vi "StoreUUTResult.vi"(8 "error in (no error)":errorcluster, 10 "Table name":string="TestResult", 11 "Result":T1 {"THD"."magnitude" format="%.2p"; "THD"."f0" format="%0.2p"; "THD"."df" format="%0.2p"}) -> (0 "error out":errorcluster={"status"=TRUE, "code"=1, "source"="DB Tools Validate Inputs.vi->DB Tools Insert Data.vi->StoreUUTResult.vi<ERR>Argument error. The table name given is blank."})   [LabVIEW 2014]
uses:
  <vilib>/addons/database/Connection.llb/DB Tools Open Connec (String).vi
  <vilib>/addons/database/NI_Database_API.lvlib
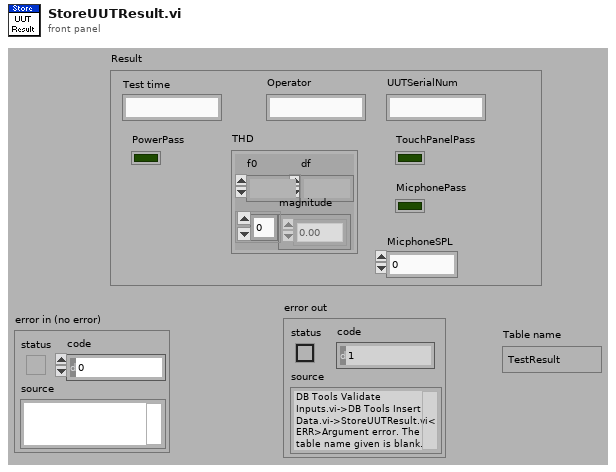
[diagram p1: front panel]
types:
  T1 = cluster{"Test time":string, "Operator":string, "UUTSerialNum":string, "PowerPass":bool, "THD":cluster{"f0":dbl, "df":dbl, "magnitude":dbl[]}, "TouchPanelPass":bool, "MicphonePass":bool, "MicphoneSPL":dbl}
  T2 = typedef "NI_Database_API.lvlib/Conn ObjectReference.ctl" = refnum<k1>
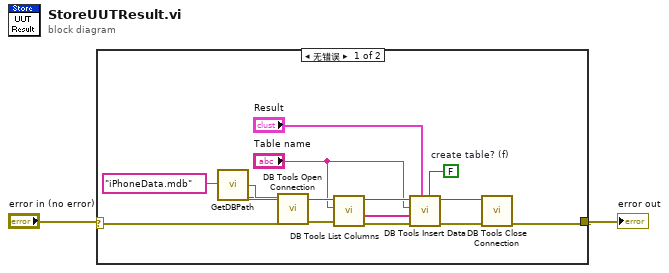
[diagram p0: block diagram]
diagram:
  n1 = case shown="无错误" "error in (no error)" {
    selector: "error in (no error)" -> [w12 w17]
    tunnel: [w11 w17] -> w1
    frame No Error {
      w10 = FALSE  # create table? (f)
      n2 = call "GetDBPath.vi"("Filename"="iPhoneData.mdb") -> ("Connection"=w14:string)
      n3 = call-poly <vilib>:"DB Tools Open Connection.vi"("error in (no error)"=w12, "connection information"=w14) -> ("error out"=w7:errorcluster, "connection reference"=w8:T2)  [unwired: 6 in]
      n4 = call <vilib>:"DB Tools List Columns.vi"("error in (no error)"=w7, "table"="Table name", "connection reference"=w8) -> ("error out"=w5:errorcluster, "columns"=w4:string[], "connection reference out"=w6:T2)  [unwired: 1 in, 1 out]
      n5 = call <vilib>:"DB Tools Insert Data.vi"("create table? (F)"=w10, "data"="Result", "error in (no error)"=w5, "columns"=w4, "table"="Table name", "connection reference"=w6) -> ("error out"=w15:errorcluster, "connection reference out"=w16:T2)  [unwired: 4 in]
      n6 = call <vilib>:"DB Tools Close Connection.vi"("error in (no error)"=w15, "connection reference"=w16) -> ("error out"=w11:errorcluster)  [unwired: 5 in]
    }
    frame Error {
    }
  }
  "error out" <- w1
